vi "RP Demo Client.vi"(8 "Error In":errorcluster, 11 "VISA resource name":refnum<visa-resource-name>="RP100") -> (0 "Error Out":errorcluster)   [LabVIEW 2016]
panel:
  out "FPGA bitfile tag":u16
  out "IDN response":u32=1 format="0x%x (%d)"
  in  "bytes to read":i32=4
  in  "Command":u64=1
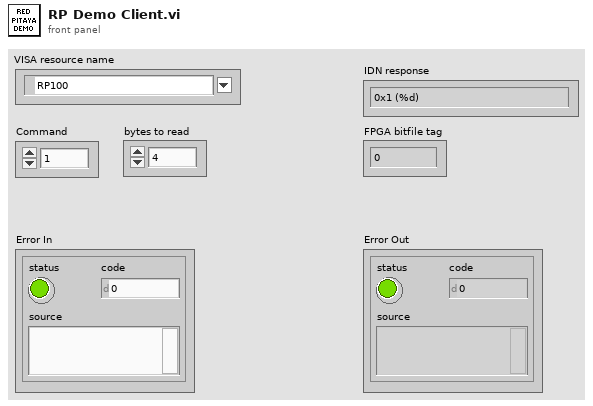
[diagram p1: front panel]
types:
  T1 = enum16{"big-endian, network order", "native, host order", "little-endian"}
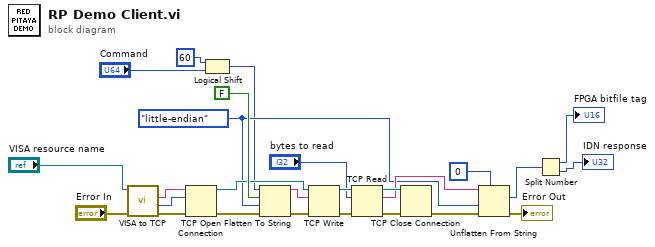
[diagram p0: block diagram]
diagram:
  w9 = T1."little-endian" ("byte order (0:big-endian, network order)")
  n1 = call "VISA to TCP.vi"("Error In"="Error In", "VISA resource name"="VISA resource name") -> ("Error Out"=w24:errorcluster, "Port"=w22:u16, "Hostname"=w23:string)  [unwired: 6 in, 1 out]
  n2 = TCP Open Connection(address=w23, remote port or service name=w22, error in (no error)=w24) -> (connection ID=w18:refnum<k5>, error out=w20:errorcluster)  [unwired: 2 in]
  n3 = Logical Shift(y=i16 60, x="Command") -> (x << y=w3:u64)
  n4 = Flatten To String(anything=w3, prepend array or string size? (T)=FALSE, byte order (0:big-endian, network order)=w9, error in (no error)=w20) -> (data string=w17:string, error out=w19:errorcluster)  [unwired: 1 out]
  n5 = TCP Write(connection ID=w18, data in=w17, error in (no error)=w19) -> (connection ID out=w15:refnum<k5>, error out=w16:errorcluster)  [unwired: 1 in, 1 out]
  n6 = TCP Read(connection ID=w15, bytes to read="bytes to read", error in (no error)=w16) -> (connection ID out=w12:refnum<k5>, data out=w11:string, error out=w13:errorcluster)  [unwired: 2 in]
  n7 = TCP Close Connection(connection ID=w12, error in (no error)=w13) -> (error out=w10:errorcluster)  [unwired: 1 in, 1 out]
  n8 = Unflatten From String(type=u32 0, binary string=w11, byte order (0:big-endian, network order)=w9, error in (no error)=w10) -> (value=w7:u32, error out=→"Error Out":errorcluster)  [unwired: 1 in, 1 out]
  n9 = Split Number(x=w7) -> (hi(x)=→"FPGA bitfile tag":u16, lo(x)=→"IDN response":u16)
